vi "Packet_decode_ByteI8.vi"(9 "StartByte":i32, 11 "RawData":u8[](array[numeric])) -> (1 "NextByte":i32, 3 "Int8_Value":i8)   [LabVIEW 2019, in "PhotonVisionLib.lvlib"]
doc: "Decode (or strip out) an unsigned byte from an array of bytes. No conversion or decoding is actually done, the memory is just copied, and the value is cast to the correct type.\n\nInputs\n - RawData -- Array of bytes containing the data to be extracted.\n - StartByte -- The starting byte number (the first byte starts at 0)\n\nOutputs\n - Int8_Value -- Byte in the form of an INT 8 value.\n - NextByte -- The starting byte index for the next value (regardless of type)."
uses:
  PhotonVisionLib.lvlib
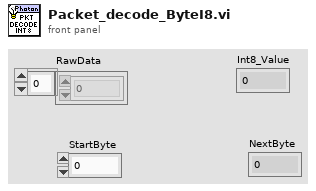
[diagram p1: front panel]
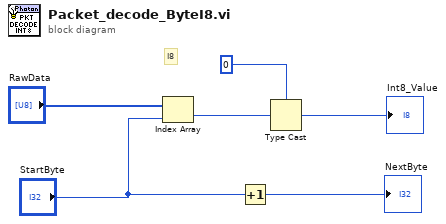
[diagram p0: block diagram]
diagram:
  # "I8"
  n1 = Index Array(array="RawData", index="StartByte") -> (element=w3:u8)
  n2 = Increment(x="StartByte") -> (x+1=→"NextByte":i32)
  n3 = Type Cast(type=i8 0, x=w3) -> (*(type *) &x=→"Int8_Value":i8)
